vi "Gen - Spreadsheet to Array.vi"(8 "Error In":errorcluster, 11 "Data in":string[](array[string])) -> (0 "Error Out":errorcluster, 3 "Data out":string[][](array[string]))   [LabVIEW 2020]
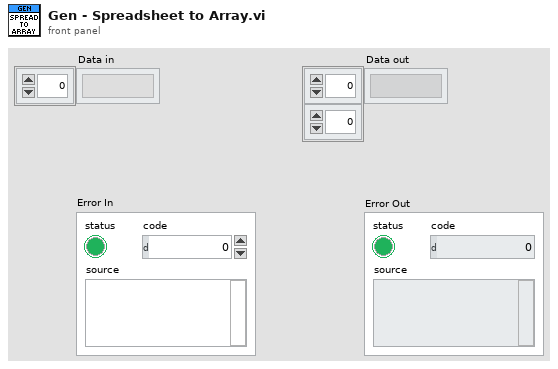
[diagram p1: front panel]
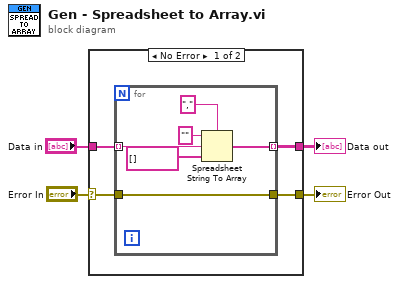
[diagram p0: block diagram]
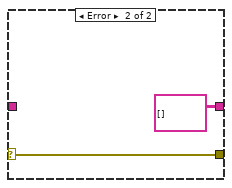
[diagram p2: hidden frame]
diagram:
  n1 = case shown="No Error" "Error In" {
    selector: "Error In" -> [w8 w16]
    tunnel: "Data in" -> [w6 _]
    tunnel: [w5 string[][] []] -> w1
    tunnel: [w7 w16] -> w3
    frame No Error {
      n2 = for {
        tunnel: w6 -> [w13] mode=indexing
        tunnel: [w9] -> w5 mode=indexing
        tunnel: [w14] -> w7
        tunnel: w8 -> [w14]
        n3 = Spreadsheet String To Array(delimiter (Tab)=",", format string="", spreadsheet string=w13, array type (2D Dbl)=string[] []) -> (array=w9:string[])
      }
    }
    frame Error {
    }
  }
  "Data out" <- w1
  "Error Out" <- w3
